vi "MeasEngine.vi"() -> (1 "XY graph visual":cluster{dbl[], dbl[]}(graph))   [LabVIEW 2026]
uses:
  <vilib>/Utility/miscctls.llb/LVRectTypeDef.ctl
  <vilib>/Utility/miscctls.llb/LVPointTypeDef.ctl
  <userlib>/Status.ctl
  <vilib>/Instr/_visa.llb/VISA Flush IO Buffer Mask.ctl
  <vilib>/Instr/_visa.llb/VISA Configure Serial Port (Instr).vi
  <vilib>/Analysis/3filter.llb/Butterworth Filter (DBL).vi
  <vilib>/measure/maspectr.llb/FFT Spectrum (Mag-Phase) for N Chan.vi
  <vilib>/measure/NI_MAPro.lvlib
  <vilib>/Analysis/NI_AALBase.lvlib
panel:
  in  "Okno osy X":dbl(slide) scale=5.0..30.0 scale format="%#_4g"
  in  "Cluster 2":T1={"Zařízení"="", "Cesta k uloženému souboru"=path "", "Vzorkovací frekvence"=enum."1000", "Record Button"=FALSE, "Stop Button"=FALSE, "A1 signál"=enum."EMG", "A2 signál"=enum."EMG", "A3 signál"=enum."EMG", "A4 signál"=enum."EMG", "A5 signál"=enum."EMG", "A6 signál"=enum."EMG", "Pin s připojeným signálem"=enum."A1"}
  in  "DO 2":bool
  in  "DO 1":bool
  out "Spectrum":cluster{"f0":dbl, "df":dbl, "magnitude":dbl[]}[](graph)
  in  "EditCluster":T2={"Horní mezní frekvence"=0.45000000000000007, "Dolní mezní frekvence"=0.0, "filter type"=enum."Lowpass", "applyFilter"=FALSE, "removeFilter"=FALSE, "undoFIlter"=FALSE} {"Horní mezní frekvence" format="%0.2f"}
  out "Waveform Graph Edit":waveform(dbl)[](graph)
  in  "DO 4":bool
  in  "DO 3":bool
  out "tdms file":refnum<k34>
  out "Ylabel and Plot name":cluster{string, string}
  out "Sample Rate Numeric":i32
  out "Consumer":i32
  out "producer":i32
  in  "error in (no error)":errorcluster
  out "Sync Stop":bool=TRUE
  # "Hz"
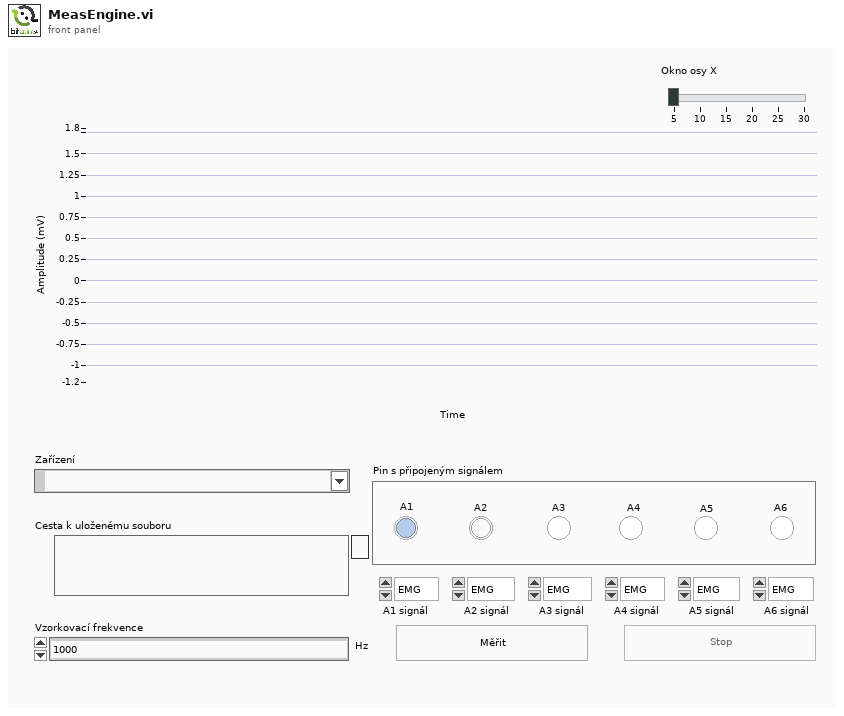
[diagram p1: front panel]
types:
  T1 = cluster{"Zařízení":refnum<visa-resource-name>, "Cesta k uloženému souboru":path, "Vzorkovací frekvence":enum16{"1", "10", "100", "1000"}, "Record Button":bool, "Stop Button":bool, "A1 signál":enum16{"EMG", "ECG", "EEG", "EDA", "ACC"}, "A2 signál":enum16{"EMG", "ECG", "EEG", "EDA", "ACC"}, "A3 signál":enum16{"EMG", "ECG", "EEG", "EDA", "ACC"}, "A4 signál":enum16{"EMG", "ECG", "EEG", "EDA", "ACC"}, "A5 signál":enum16{"EMG", "ECG", "EEG", "EDA", "ACC"}, "A6 signál":enum16{"EMG", "ECG", "EEG", "EDA", "ACC"}, "Pin s připojeným signálem":enum32{"A1", "A2", "A3", "A4", "A5", "A6"}}
  T2 = cluster{"Horní mezní frekvence":dbl, "Dolní mezní frekvence":dbl, "filter type":enum32{"Lowpass", "Highpass", "Bandpass", "Bandstop"}, "applyFilter":bool, "removeFilter":bool, "undoFIlter":bool}
  T3 = typedef "Status.ctl" = enum16{"Initialize", "Edit", "Standby", "Recording", "Exit"}
  T4 = enum16{"Always On", "Always Off", "Off While Running"}
  T5 = typedef "LVPointTypeDef.ctl" = cluster{"Horizontal":i16, "Vertical":i16}
  T6 = typedef "LVRectTypeDef.ctl" = cluster{"Left":i16, "Top":i16, "Right":i16, "Bottom":i16}
  T7 = enum8{"Enabled", "Disabled", "Disabled and Grayed Out"}
  T8 = enum16{"open", "open or create", "create or replace", "create", "open (read-only)"}
  T9 = typedef "VISA Flush IO Buffer Mask.ctl" = u16
  T10 = enum32{"Lowpass", "Highpass", "Bandpass", "Bandstop"}
  T11 = cluster{"A1 signál":enum16{"EMG", "ECG", "EEG", "EDA", "ACC"}, "A2 signál":enum16{"EMG", "ECG", "EEG", "EDA", "ACC"}, "A3 signál":enum16{"EMG", "ECG", "EEG", "EDA", "ACC"}, "A4 signál":enum16{"EMG", "ECG", "EEG", "EDA", "ACC"}, "A5 signál":enum16{"EMG", "ECG", "EEG", "EDA", "ACC"}, "A6 signál":enum16{"EMG", "ECG", "EEG", "EDA", "ACC"}}
  T12 = cluster{"Result":dbl, "Result":dbl, "Result":dbl, "Result":dbl, "Result":dbl, "Result":dbl}
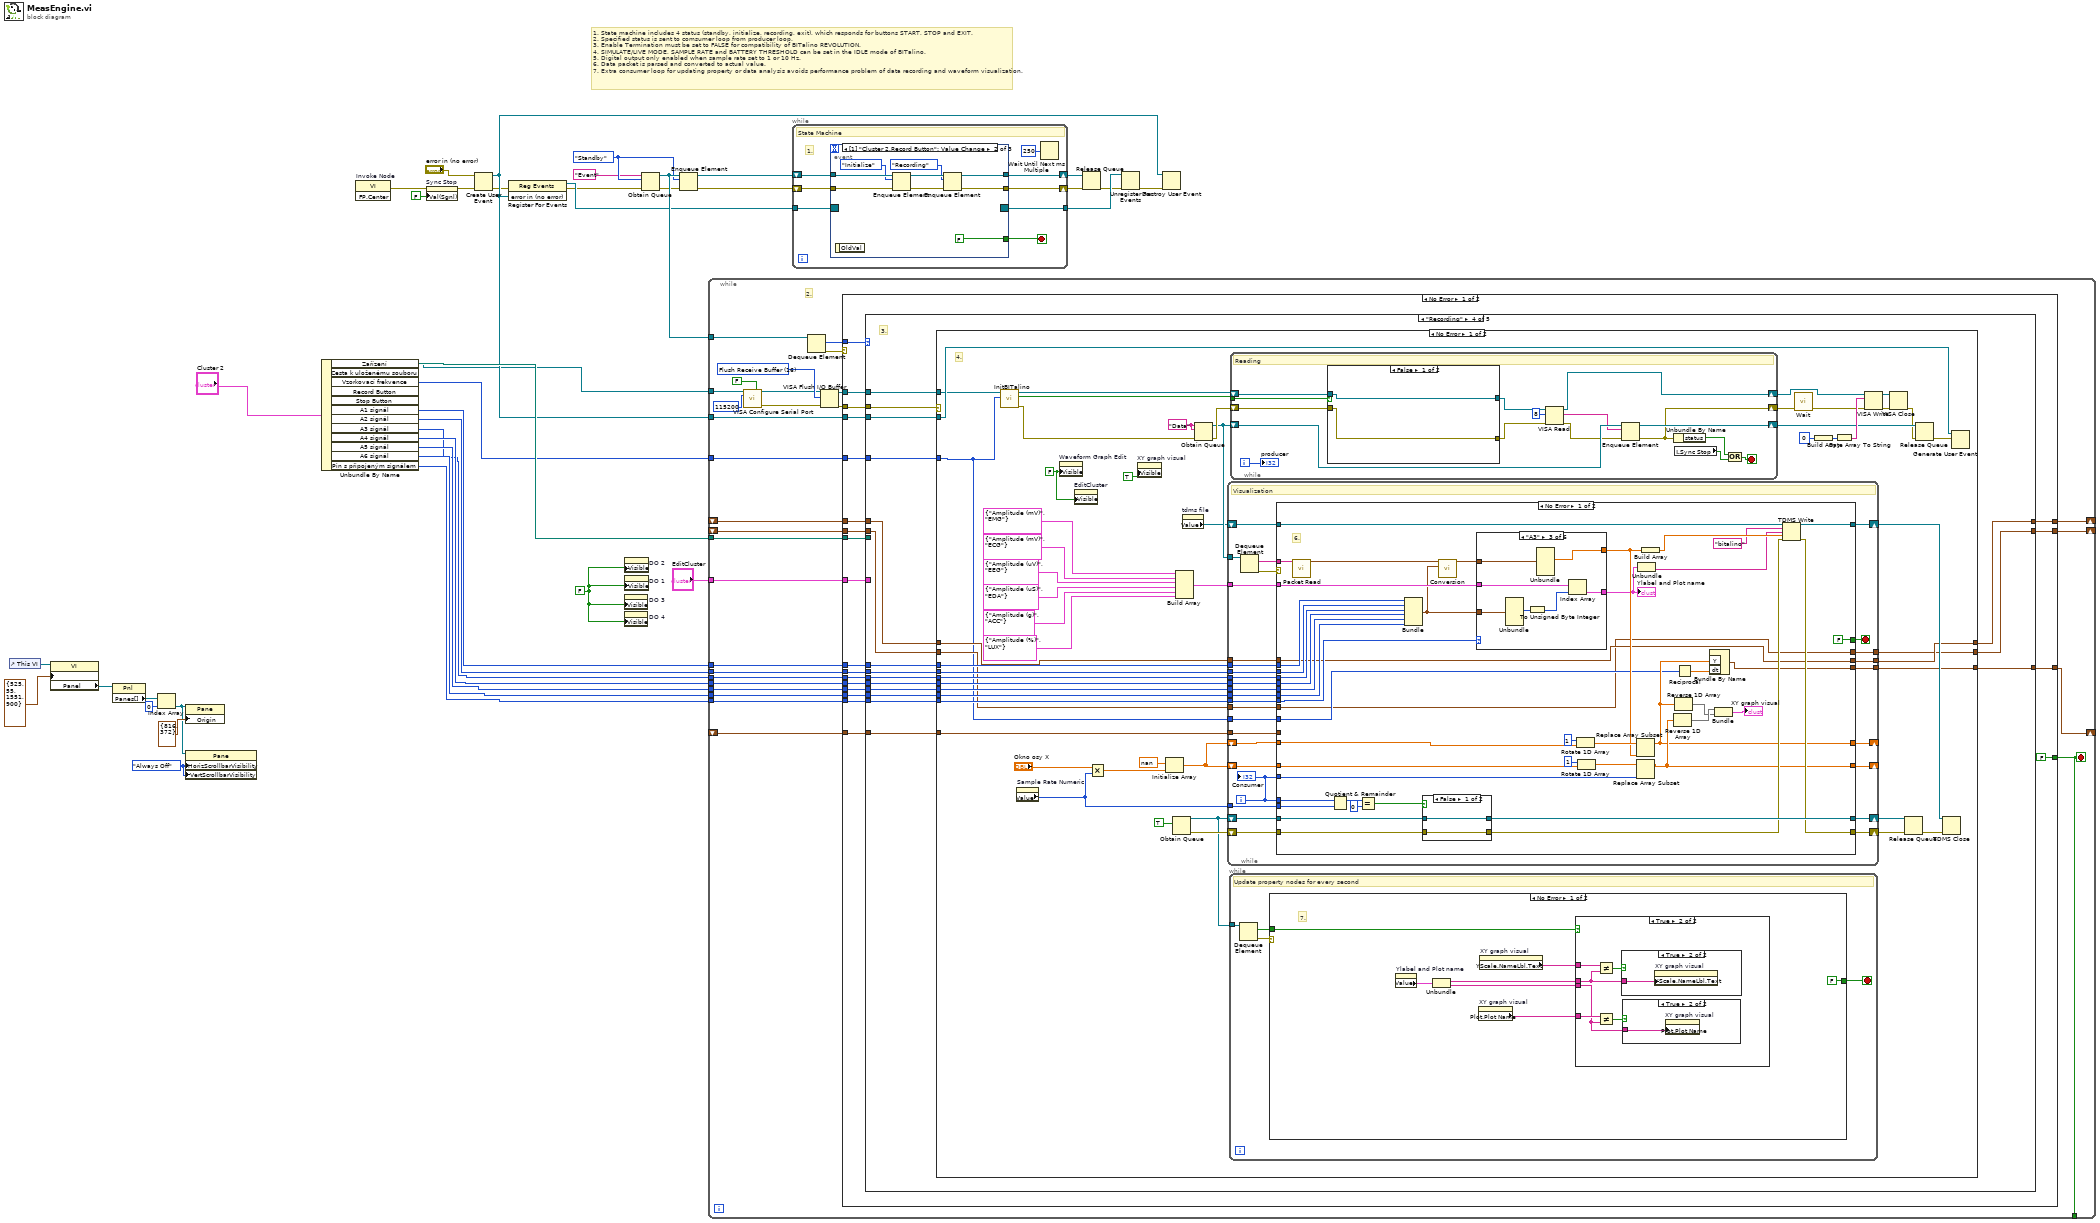
[diagram p0: block diagram]
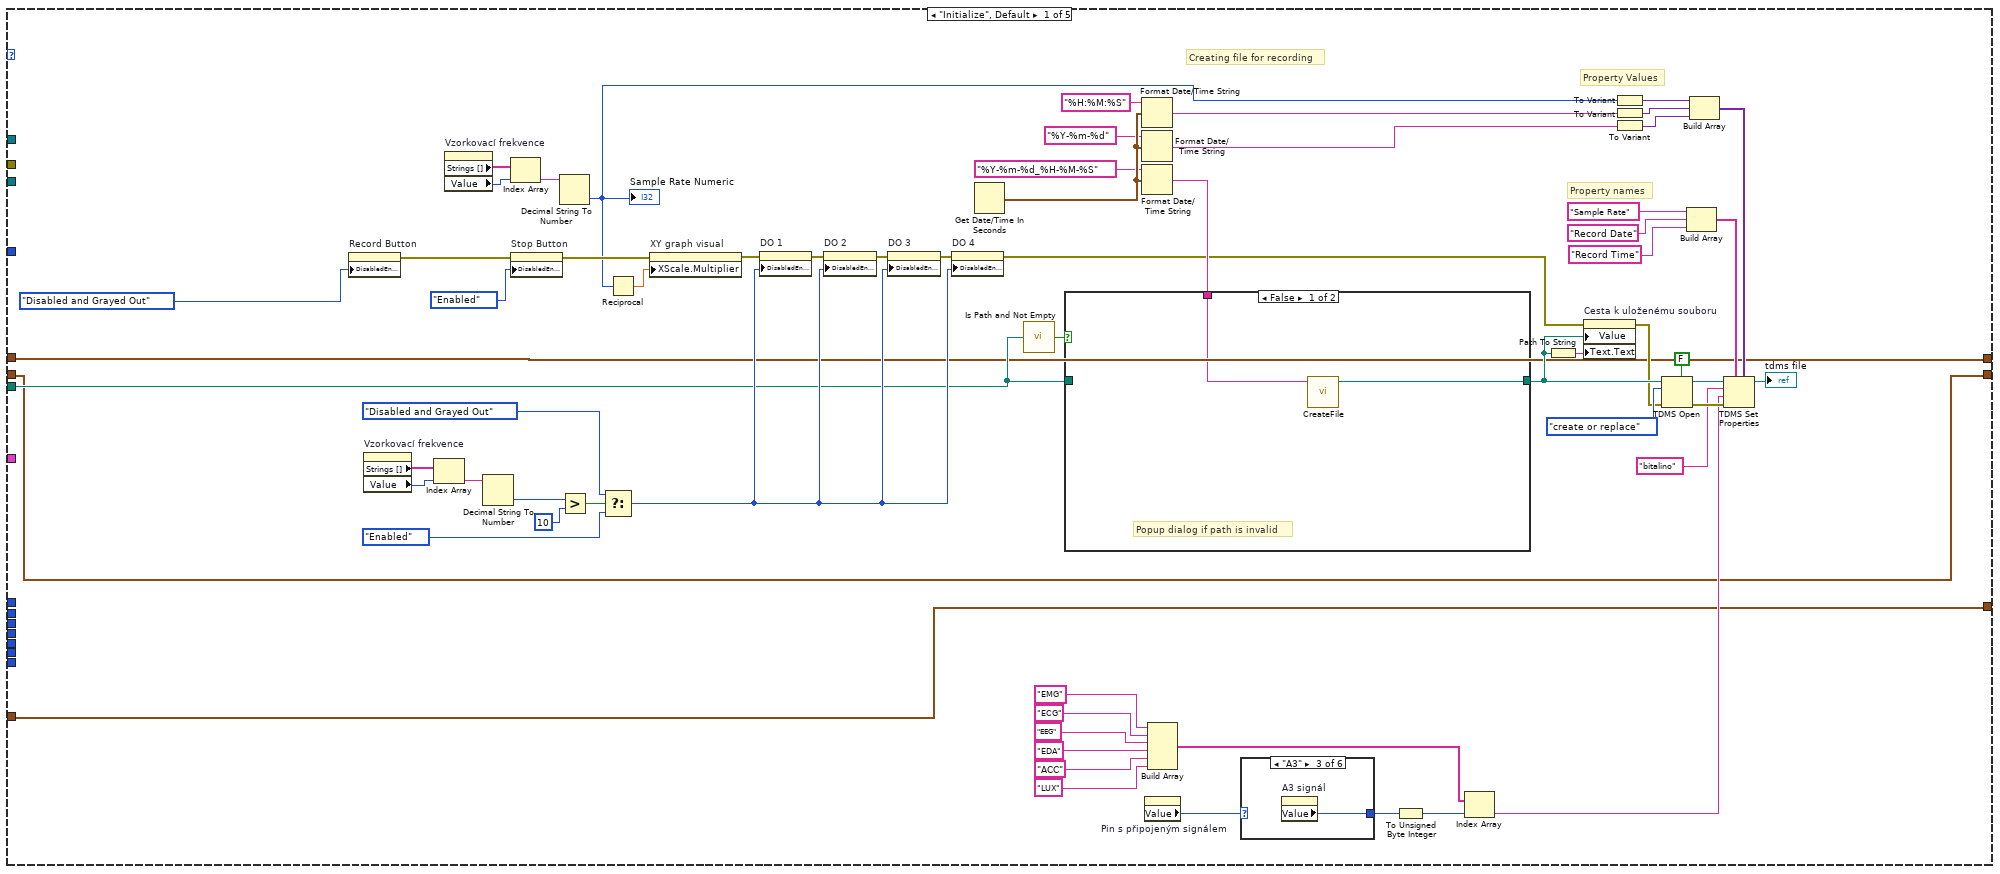
[diagram p2: hidden frame]
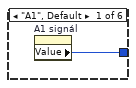
[diagram p3: hidden frame]
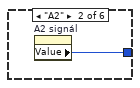
[diagram p4: hidden frame]
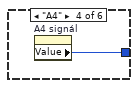
[diagram p5: hidden frame]
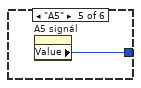
[diagram p6: hidden frame]
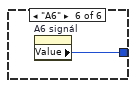
[diagram p7: hidden frame]
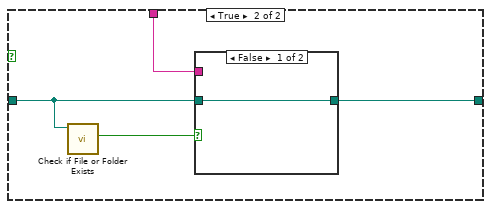
[diagram p8: hidden frame]
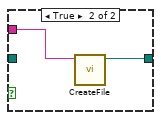
[diagram p9: hidden frame]
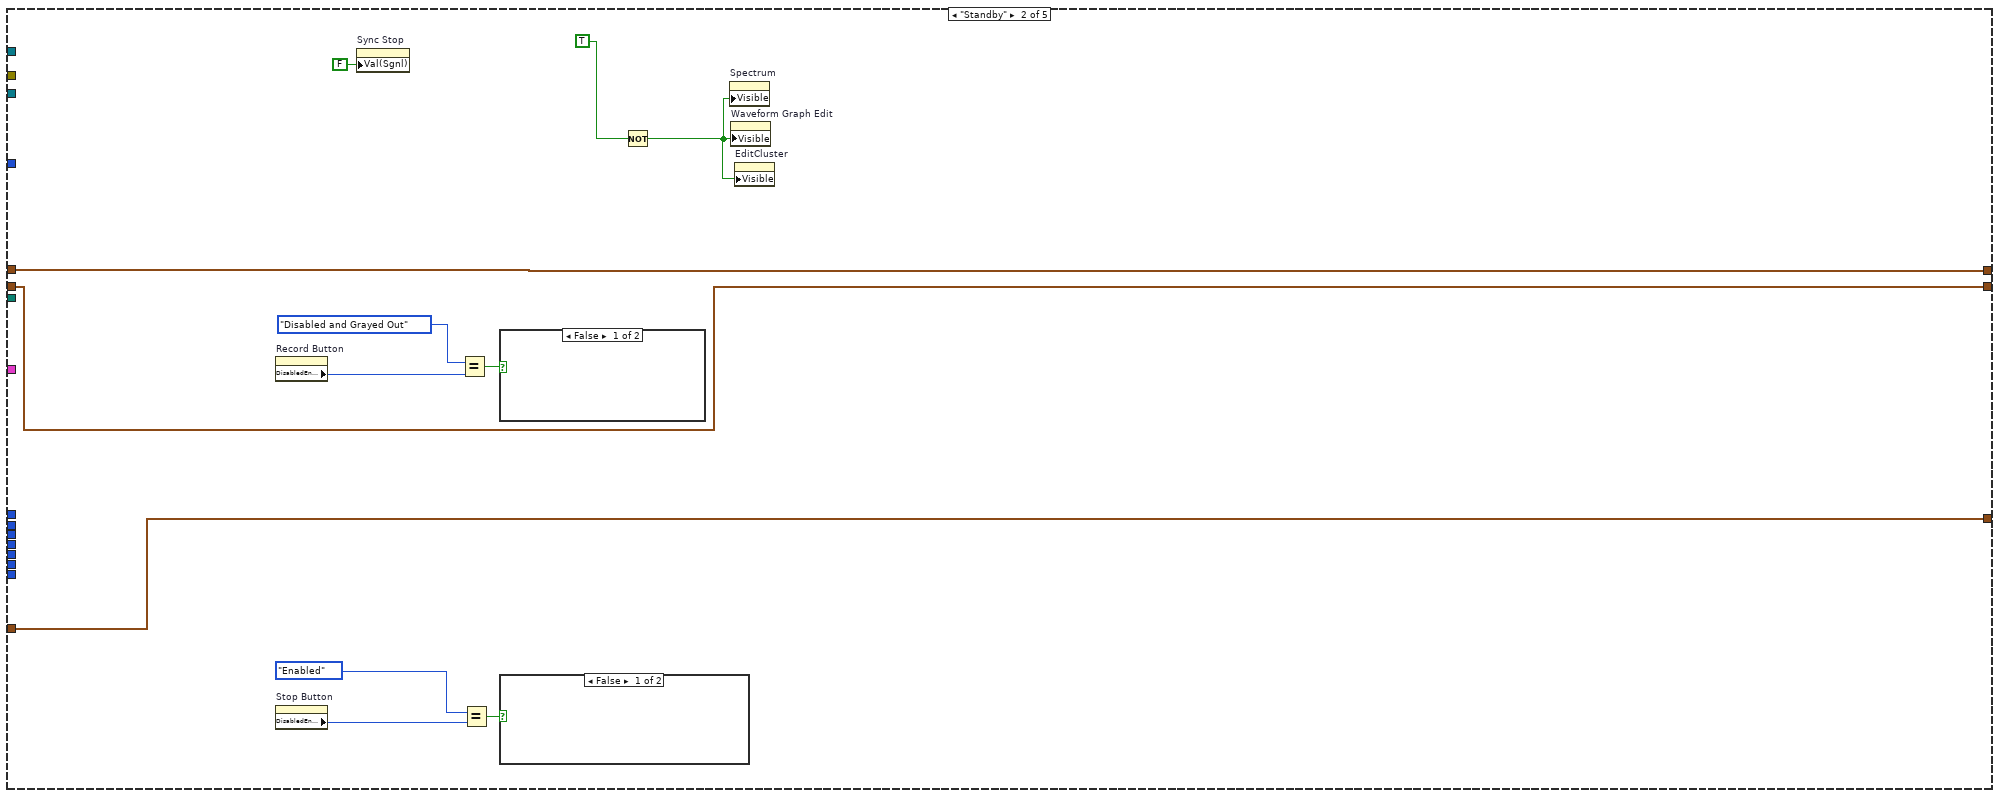
[diagram p10: hidden frame]
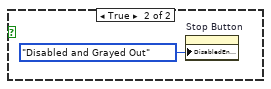
[diagram p11: hidden frame]
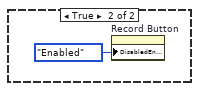
[diagram p12: hidden frame]
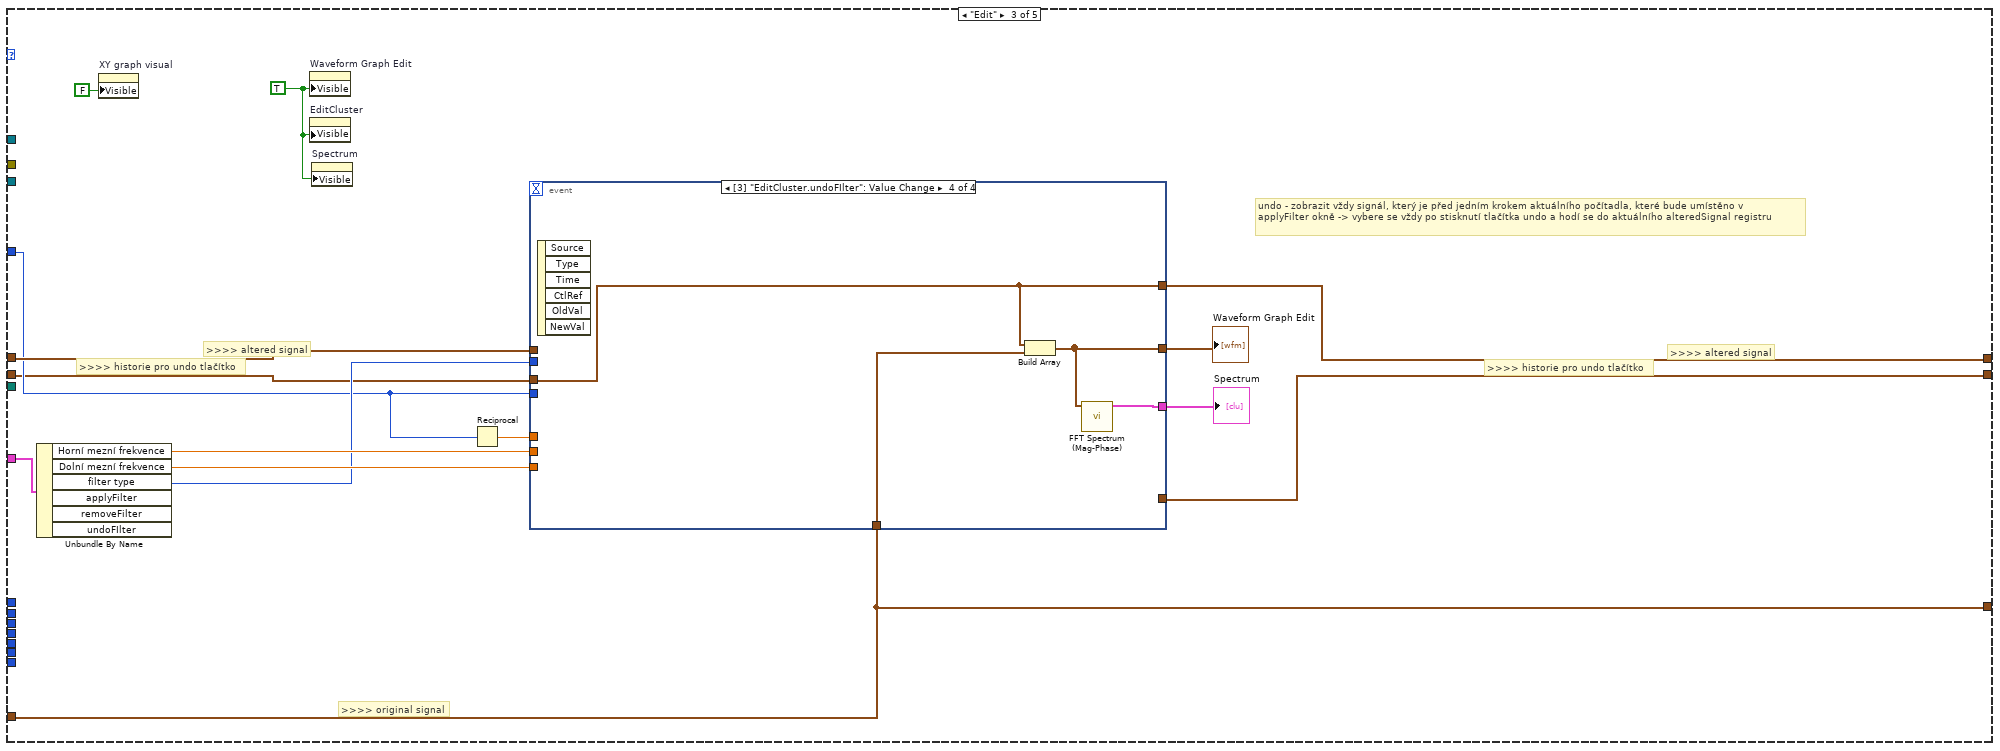
[diagram p13: hidden frame]
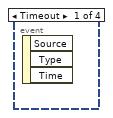
[diagram p14: hidden frame]
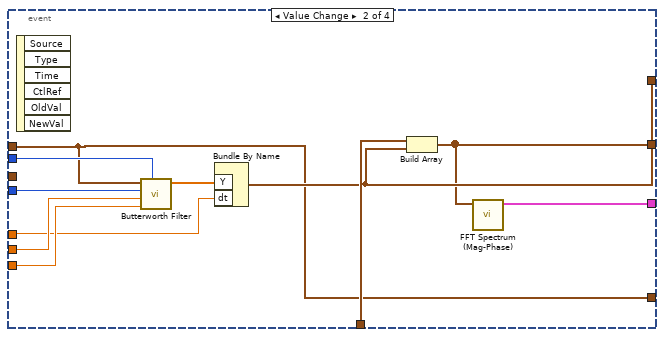
[diagram p15: hidden frame]
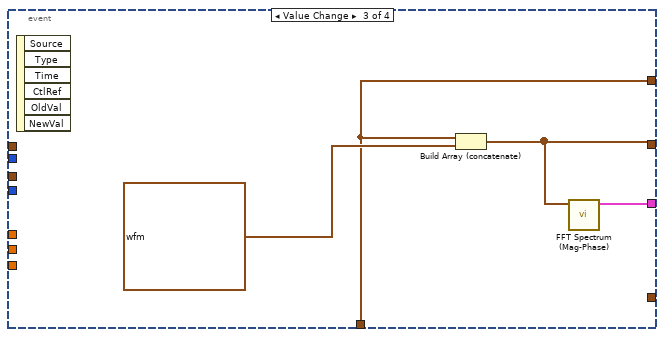
[diagram p16: hidden frame]
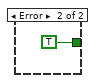
[diagram p20: hidden frame]
diagram:
  w5 = FALSE
  w3 = Status."Standby" ("Enum")
  w33 = T4."Always Off" ("Horizontal Scrollbar Visibility")
  # "1. State machine includes 4 status (standby, initialize, recording, exit), which responds for buttons START, STOP and EXIT.\n2. Specified status is sent to comsumer loop from producer loop.\n3. Enable Termination must be set to FALSE for compatibility of BITalino REVOLUTION.\n4. SIMULATE/LIVE MODE, SAMPLE RATE and BATTERY THRESHOLD can be set in the IDLE mode of BITalino.\n5. Digital output only enabled when sample rate set to 1 or 10 Hz.\n6. Data packet is parsed and converted to actual value.\n7. Extra consumer loop for updating property or data analysis avoids performance problem of data recording and waveform visualization."
  n1 = control-ref of="This VI"() -> (w40:refnum<vi>)
  n2 = property class="VI"(reference=w40, "Front Panel.WinBounds"=T6 {"Left"=525, "Top"=55, "Right"=1551, "Bottom"=900} ("Front Panel Window:Window Bounds")) -> ("Panel"=w38:refnum<vi>)  [unwired: 1 in, 2 out]
  n3 = property class="Pnl"(reference=w38) -> ("Panes[]"=w37:refnum<vi>[])  [unwired: 1 in, 2 out]
  n4 = Index Array(array=w37, index=0) -> (element=w34:refnum<vi>)
  n5 = property class="Pane"(reference=w34, "Origin"=T5 {"Horizontal"=816, "Vertical"=372}) -> ()  [unwired: 1 in, 2 out]
  n6 = property class="Pane"(reference=w34, "HorizScrollbarVisibility"=w33, "VertScrollbarVisibility"=w33) -> ()  [unwired: 1 in, 2 out]
  n7 = Unbundle By Name("Cluster 2") -> ("Zařízení"=w1:refnum<visa-resource-name>, "Cesta k uloženému souboru"=w30:path, "Vzorkovací frekvence"=w22:enum16{"1", "10", "100", "1000"}, "A1 signál"=w23:enum16{"EMG", "ECG", "EEG", "EDA", "ACC"}, "A2 signál"=w24:enum16{"EMG", "ECG", "EEG", "EDA", "ACC"}, "A3 signál"=w25:enum16{"EMG", "ECG", "EEG", "EDA", "ACC"}, "A4 signál"=w26:enum16{"EMG", "ECG", "EEG", "EDA", "ACC"}, "A5 signál"=w27:enum16{"EMG", "ECG", "EEG", "EDA", "ACC"}, "A6 signál"=w28:enum16{"EMG", "ECG", "EEG", "EDA", "ACC"}, "Pin s připojeným signálem"=w29:enum32{"A1", "A2", "A3", "A4", "A5", "A6"})  [unwired: 2 out]
  n8 = invoke on="Invoke Node" class="VI" method="FP.Center"() -> (error out=w20:errorcluster)  [unwired: 3 in, 2 out]
  n9 = property on="Sync Stop" class="Bool (strict)"(error in=w20, "Val(Sgnl)"=FALSE ("Value (Signaling)")) -> (error out=w11:errorcluster)  [unwired: 1 in, 1 out]
  n10 = Create User Event(user event datatype="error in (no error)", error in=w11) -> (user event=w19:refnum<user-event>, error out=w12:errorcluster)
  n11 = register-events(error in=w12, w19) -> (reference out=w14:refnum<event-registration>, error out=w13:errorcluster)  [unwired: 1 in]
  n12 = property on="DO 3" class="Bool (strict)"("Visible"=w5) -> ()  [unwired: 2 in, 2 out]
  n13 = property on="DO 4" class="Bool (strict)"("Visible"=w5) -> ()  [unwired: 2 in, 2 out]
  n14 = property on="DO 2" class="Bool (strict)"("Visible"=w5) -> ()  [unwired: 2 in, 2 out]
  n15 = property on="DO 1" class="Bool (strict)"("Visible"=w5) -> ()  [unwired: 2 in, 2 out]
  n16 = Obtain Queue(name (unnamed)="Event", element data type=w3, error in (no error)=w13) -> (queue out=w21:refnum<queue>, error out=w8:errorcluster)  [unwired: 2 in, 1 out]
  n17 = Enqueue Element(queue=w21, element=w3, error in (no error)=w8) -> (queue out=w10:refnum<queue>, error out=w9:errorcluster)  [unwired: 1 in, 1 out]
  n18 = while {
    tunnel: w21 -> [w69]
    tunnel: w19 -> [w49]
    tunnel: w22 -> [w66]
    tunnel: [w65] -> _
    tunnel: w23 -> [w64]
    tunnel: w24 -> [w63]
    tunnel: w25 -> [w62]
    tunnel: w26 -> [w61]
    tunnel: w27 -> [w60]
    tunnel: w28 -> [w59]
    tunnel: w29 -> [w58]
    tunnel: w30 -> [w57]
    shift-right: [w56] -> _
    shift-left: _ -> [w55]
    tunnel: "EditCluster" -> [w54]
    shift-right: [w53] -> _
    shift-left: _ -> [w52]
    shift-right: [w51] -> _
    shift-left: _ -> [w50]
    tunnel: w1 -> [w45]
    stop <- w65 stop-if-true
    w46 = T9 16 items=["Flush Receive Buffer"=16, "Write Transmit Buffer to Device"=32, "Flush Receive Buffer (No I/O)"=64, "Flush Transmit Buffer"=128] ("Mask")
    # "2."
    n19 = call-poly "VISA Configure Serial Port"("VISA resource name"=w45, "Enable Termination\nChar (T)"=FALSE ("Enable Termination\nChar (T)"), "baud rate (9600)"=u32 115200) -> ("VISA resource name out"=w42:refnum<visa-resource-name>, "error out"=w41:errorcluster)  [unwired: 11 in]
    n20 = Dequeue Element(queue=w69) -> (element=w68:T3, error out=w67:errorcluster)  [unwired: 2 in, 2 out]
    n21 = VISA Flush I/O Buffer(VISA resource name=w42, mask (16)=w46, error in (no error)=w41) -> (VISA resource name out=w47:refnum<visa-resource-name>, error out=w48:errorcluster)
    n22 = case shown="No Error" w67 {
      tunnel: w68 -> [w88 _]
      tunnel: [FALSE TRUE] -> w65
      tunnel: w66 -> [w89 _]
      tunnel: w64 -> [w87 _]
      tunnel: w63 -> [w86 _]
      tunnel: w62 -> [w85 _]
      tunnel: w61 -> [w84 _]
      tunnel: w60 -> [w83 _]
      tunnel: w59 -> [w82 _]
      tunnel: w58 -> [w81 _]
      tunnel: w57 -> [w80 _]
      tunnel: [w79 w484] -> w56
      tunnel: w55 -> [w78 w484]
      tunnel: w54 -> [w77 _]
      tunnel: [w76 w483] -> w53
      tunnel: w52 -> [w75 w483]
      tunnel: [w74 w482] -> w51
      tunnel: w50 -> [w73 w482]
      tunnel: w49 -> [w72 _]
      tunnel: w48 -> [w71 _]
      tunnel: w47 -> [w70 _]
      frame No Error {
        n23 = case shown="\"Recording\"" w88 {
          tunnel: w89 -> [_ _ w189 w233 _]
          tunnel: w87 -> [_ _ _ w232 _]
          tunnel: w86 -> [_ _ _ w231 _]
          tunnel: w85 -> [_ _ _ w230 _]
          tunnel: w84 -> [_ _ _ w229 _]
          tunnel: w83 -> [_ _ _ w228 _]
          tunnel: w82 -> [_ _ _ w227 _]
          tunnel: w81 -> [_ _ _ w226 _]
          tunnel: w80 -> [w95 _ _ _ _]
          tunnel: [w94 w173 w186 w225 w479] -> w79
          tunnel: w78 -> [w94 w173 w186 w224 w479]
          tunnel: w77 -> [_ _ w196 _ _]
          tunnel: [w93 w169 w185 w223 w478] -> w76
          tunnel: w75 -> [w93 w169 w194 w222 w478]
          tunnel: [w92 w171 w184 w221 w477] -> w74
          tunnel: w73 -> [w92 w171 w183 w220 w477]
          tunnel: w72 -> [_ _ _ w219 _]
          tunnel: w71 -> [_ _ _ w218 _]
          tunnel: w70 -> [_ _ _ w217 _]
          frame "Initialize", Default {
            # "Creating file for recording"
            # "Property Values"
            # "Property names"
            n24 = property on="Record Button" class="Bool"("DisabledEnum"=T7."Disabled and Grayed Out" ("Disabled")) -> (error out=w91:errorcluster)  [unwired: 2 in, 1 out]
            n25 = property on="Vzorkovací frekvence" class="Enum (strict)"() -> ("Strings []"=w113:string[], "Value"=w112:enum16{"1", "10", "100", "1000"})  [unwired: 2 in, 2 out]
            n26 = Index Array "Index Array"(array=w113, index=w112) -> (element=w111:string)
            n27 = property on="Vzorkovací frekvence" class="Enum (strict)"() -> ("Strings []"=w152:string[], "Value"=w151:enum16{"1", "10", "100", "1000"})  [unwired: 2 in, 2 out]
            n28 = Decimal String To Number(string=w111) -> (number=w110:i32)  [unwired: 2 in, 1 out]
            n29 = Index Array(array=w152, index=w151) -> (element=w150:string)
            n30 = property on="Stop Button" class="Bool"(error in=w91, "DisabledEnum"=T7."Enabled" ("Disabled")) -> (error out=w149:errorcluster)  [unwired: 1 in, 1 out]
            n31 = Decimal String To Number(string=w150) -> (number=w122:i32)  [unwired: 2 in, 1 out]
            "Sample Rate Numeric" <- w122
            n32 = Greater?(x=w110, y=10) -> (0:w118:bool)
            n33 = Select(t=T7."Disabled and Grayed Out" ("Disabled"), s=w118, f=T7."Enabled" ("Disabled")) -> (s? t:f=w121:T7)
            n34 = Reciprocal(x=w122) -> (1/x=w148:dbl)
            n35 = property on="XY graph visual" class="XYGraph (strict)"(error in=w149, "XScale.Multiplier"=w148) -> (error out=w109:errorcluster)  [unwired: 1 in, 1 out]
            n36 = property on="DO 1" class="Bool (strict)"(error in=w109, "DisabledEnum"=w121) -> (error out=w116:errorcluster)  [unwired: 1 in, 1 out]
            n37 = property on="DO 2" class="Bool (strict)"(error in=w116, "DisabledEnum"=w121) -> (error out=w115:errorcluster)  [unwired: 1 in, 1 out]
            n38 = property on="DO 3" class="Bool (strict)"(error in=w115, "DisabledEnum"=w121) -> (error out=w114:errorcluster)  [unwired: 1 in, 1 out]
            n39 = property on="DO 4" class="Bool (strict)"(error in=w114, "DisabledEnum"=w121) -> (error out=w108:errorcluster)  [unwired: 1 in, 1 out]
            n40 = Get Date/Time In Seconds() -> (seconds since 1Jan1904=w138:timestamp)
            n41 = call <vilib>:"Is Path and Not Empty.vi"("path"=w95) -> ("Is Path and Not Empty?"=w130:bool)  [unwired: 4 in]
            n42 = Format Date/Time String(time format string (%c)="%H:%M:%S", seconds (now)=w138) -> (date/time string=w143:string)  [unwired: 1 in]
            n43 = Format Date/Time String(time format string (%c)="%Y-%m-%d", seconds (now)=w138) -> (date/time string=w144:string)  [unwired: 1 in]
            n44 = Format Date/Time String(time format string (%c)="%Y-%m-%d_%H-%M-%S", seconds (now)=w138) -> (date/time string=w134:string)  [unwired: 1 in]
            n45 = case shown="False" w130 {
              tunnel: [w160 w163] -> w127
              tunnel: w95 -> [_ w162]
              tunnel: w134 -> [w161 w164]
              frame False {
                # "Popup dialog if path is invalid"
                n46 = call "CreateFile.vi"("date/time string"=w161) -> ("appended path"=w160:path)  [unwired: 10 in]
              }
              frame True {
                n47 = call <vilib>:"Check if File or Folder Exists.vi"("path"=w162) -> ("file or folder exists?"=w165:bool)  [unwired: 8 in, 2 out]
                n48 = case shown="False" w165 {
                  tunnel: w164 -> [_ w168]
                  tunnel: [w166 w167] -> w163
                  tunnel: w162 -> [w166 _]
                  frame False {
                  }
                  frame True {
                    n49 = call "CreateFile.vi"("date/time string"=w168) -> ("appended path"=w167:path)  [unwired: 10 in]
                  }
                }
              }
            }
            n50 = property on="Pin s připojeným signálem" class="RadioBtnsControl (strict)"() -> ("Value"=w106:enum32{"A1", "A2", "A3", "A4", "A5", "A6"})  [unwired: 2 in, 2 out]
            n51 = Build Array("EMG", "ECG", "EEG", "EDA", "ACC", "LUX") -> (w97:string[])
            n52 = case shown="\"A3\"" w106 {
              tunnel: [w154 w155 w156 w157 w158 w159] -> w99
              frame "A1", Default {
                n53 = property on="A1 signál" class="Enum (strict)"() -> ("Value"=w154:enum16{"EMG", "ECG", "EEG", "EDA", "ACC"})  [unwired: 2 in, 2 out]
              }
              frame "A2" {
                n54 = property on="A2 signál" class="Enum (strict)"() -> ("Value"=w155:enum16{"EMG", "ECG", "EEG", "EDA", "ACC"})  [unwired: 2 in, 2 out]
              }
              frame "A3" {
                n55 = property on="A3 signál" class="Enum (strict)"() -> ("Value"=w156:enum16{"EMG", "ECG", "EEG", "EDA", "ACC"})  [unwired: 2 in, 2 out]
              }
              frame "A4" {
                n56 = property on="A4 signál" class="Enum (strict)"() -> ("Value"=w157:enum16{"EMG", "ECG", "EEG", "EDA", "ACC"})  [unwired: 2 in, 2 out]
              }
              frame "A5" {
                n57 = property on="A5 signál" class="Enum (strict)"() -> ("Value"=w158:enum16{"EMG", "ECG", "EEG", "EDA", "ACC"})  [unwired: 2 in, 2 out]
              }
              frame "A6" {
                n58 = property on="A6 signál" class="Enum (strict)"() -> ("Value"=w159:enum16{"EMG", "ECG", "EEG", "EDA", "ACC"})  [unwired: 2 in, 2 out]
              }
            }
            n59 = To Unsigned Byte Integer(number=w99) -> (unsigned 8bit integer=w98:u8)
            n60 = Index Array(array=w97, index=w98) -> (element=w96:string)
            n61 = Path To String(path=w127) -> (string=w128:string)
            n62 = property on="Cesta k uloženému souboru" class="Path"(error in=w108, "Value"=w127, "Text.Text"=w128) -> (error out=w126:errorcluster)  [unwired: 1 in, 1 out]
            n63 = To Variant(anything=w122) -> (Variant=w142:variant)
            n64 = To Variant(anything=w143) -> (Variant=w145:variant)
            n65 = To Variant(anything=w144) -> (Variant=w146:variant)
            n66 = TDMS Open(5:FALSE ("create index file? (T)"), 8:w126, 10:T8."create or replace" ("operation (0:open)"), 11:w127) -> (0:w133:errorcluster, 3:w132:refnum<k34>)  [unwired: 3 in]
            n67 = Build Array("Sample Rate", "Record Date", "Record Time") -> (w141:string[])
            n68 = Build Array(w142, w145, w146) -> (w147:variant[])
            n69 = TDMS Set Properties(5:w147, 7:w141, 8:w133, 9:w96, 10:"bitalino", 11:w132) -> (3:→"tdms file":refnum<k34>)  [unwired: 3 out]
          }
          frame "Standby" {
            n70 = property on="Record Button" class="Bool"() -> ("DisabledEnum"=w179:T7)  [unwired: 2 in, 2 out]
            n71 = property on="Stop Button" class="Bool"() -> ("DisabledEnum"=w176:T7)  [unwired: 2 in, 2 out]
            n72 = property on="Sync Stop" class="Bool (strict)"("Val(Sgnl)"=FALSE ("Value (Signaling)")) -> ()  [unwired: 2 in, 2 out]
            n73 = Equal?(x=T7."Disabled and Grayed Out" ("Disabled"), y=w179) -> (x = y?=w178:bool)
            n74 = Equal?(x=T7."Enabled" ("Disabled"), y=w176) -> (x = y?=w175:bool)
            n75 = case shown="False" w178 {
              frame False {
              }
              frame True {
                n76 = property on="Record Button" class="Bool"("DisabledEnum"=T7."Enabled" ("Disabled")) -> ()  [unwired: 2 in, 2 out]
              }
            }
            n77 = case shown="False" w175 {
              frame False {
              }
              frame True {
                n78 = property on="Stop Button" class="Bool"("DisabledEnum"=T7."Disabled and Grayed Out" ("Disabled")) -> ()  [unwired: 2 in, 2 out]
              }
            }
            n79 = Not(x=TRUE ("Visible")) -> (.not. x?=w172:bool)
            n80 = property on="Spectrum" class="WFGraph (strict)"("Visible"=w172) -> ()  [unwired: 2 in, 2 out]
            n81 = property on="Waveform Graph Edit" class="WFGraph (strict)"("Visible"=w172) -> ()  [unwired: 2 in, 2 out]
            n82 = property on="EditCluster" class="Clust"("Visible"=w172) -> ()  [unwired: 2 in, 2 out]
          }
          frame "Edit" {
            w195 = TRUE ("Visible")
            # ">>>> altered signal"
            # ">>>> historie pro undo tlačítko"
            # ">>>> historie pro undo tlačítko"
            # "undo - zobrazit vždy signál, který je před jedním krokem aktuálního počítadla, které bude umístěno v \napplyFilter okně -> vybere se vždy po stisknutí tlačítka undo a hodí se do aktuálního alteredSignal registru"
            # ">>>> altered signal"
            # ">>>> original signal"
            n83 = Unbundle By Name(w196) -> ("Horní mezní frekvence"=w192:dbl, "Dolní mezní frekvence"=w191:dbl, "filter type"=w190:T10)  [unwired: 3 out]
            n84 = property on="XY graph visual" class="XYGraph (strict)"("Visible"=FALSE) -> ()  [unwired: 2 in, 2 out]
            n85 = property on="Waveform Graph Edit" class="WFGraph (strict)"("Visible"=w195) -> ()  [unwired: 2 in, 2 out]
            n86 = property on="EditCluster" class="Clust"("Visible"=w195) -> ()  [unwired: 2 in, 2 out]
            n87 = property on="Spectrum" class="WFGraph (strict)"("Visible"=w195) -> ()  [unwired: 2 in, 2 out]
            n88 = Reciprocal(x=w189) -> (1/x=w193:dbl)
            n89 = event shown="[3] \"EditCluster.undoFIlter\": Value Change" {
              selector: _ -> [_ _ _ _]
              dyn-events: _ -> [_ _ _ _]
              timeout: _ -> [_ _ _ _]
              tunnel: w186 -> [_ w207 w209 w215]
              tunnel: [_ w206 w209 w216] -> w185
              tunnel: w194 -> [_ w198 _ _]
              tunnel: w193 -> [_ w202 _ _]
              tunnel: w192 -> [_ w205 _ _]
              tunnel: w191 -> [_ w204 _ _]
              tunnel: w190 -> [_ w203 _ _]
              tunnel: w189 -> [_ w201 _ _]
              tunnel: [_ w200 w210 w213] -> w188
              tunnel: [_ w199 w211 w214] -> w187
              tunnel: [_ w198 _ _] -> w184
              tunnel: w183 -> [_ _ _ w216]
              event Timeout {
                n90 = event-data() -> ()  [unwired: 1 in, 3 out]
              }
              event "EditCluster.applyFilter": Value Change {
                n91 = event-data() -> ()  [unwired: 1 in, 6 out]
                n92 = call-poly <vilib>:"Butterworth Filter.vi"("filter type"=w203, "low cutoff freq: fl"=w204, "high cutoff freq: fh"=w205, "sampling freq: fs"=w201, "X"=w198) -> ("Filtered X"=w208:dbl[])  [unwired: 3 in, 1 out]
                n93 = Bundle By Name("Y"=w208, "dt"=w202) -> (w206:waveform(dbl))  [unwired: 1 in]
                n94 = Build Array(w207, w206) -> (w200:waveform(dbl)[])
                n95 = call-poly <vilib>:"FFT Spectrum (Mag-Phase).vi"("time signals"=w200) -> ("magnitudes"=w199:cluster{"f0":dbl, "df":dbl, "magnitude":dbl[]}[])  [unwired: 6 in, 4 out]
              }
              event "EditCluster.removeFilter": Value Change {
                n96 = event-data() -> ()  [unwired: 1 in, 6 out]
                n97 = Build Array (concatenate)(w209, waveform(dbl)[] [{"t0"=timestamp(-3600 s since 1904-01-01), "dt"=10000.0, "Y"=[0.0]}] ("array")) -> (w210:waveform(dbl)[])
                n98 = call-poly <vilib>:"FFT Spectrum (Mag-Phase).vi"("time signals"=w210) -> ("magnitudes"=w211:cluster{"f0":dbl, "df":dbl, "magnitude":dbl[]}[])  [unwired: 6 in, 4 out]
              }
              event "EditCluster.undoFIlter": Value Change {
                n99 = event-data() -> ()  [unwired: 1 in, 6 out]
                n100 = Build Array(w216, w215) -> (w213:waveform(dbl)[])
                n101 = call-poly <vilib>:"FFT Spectrum (Mag-Phase).vi"("time signals"=w213) -> ("magnitudes"=w214:cluster{"f0":dbl, "df":dbl, "magnitude":dbl[]}[])  [unwired: 6 in, 4 out]
              }
            }
            "Waveform Graph Edit" <- w188
            "Spectrum" <- w187
          }
          frame "Recording" {
            # "3."
            n102 = case shown="No Error" w218 {
              selector: w218 -> [_ w475]
              tunnel: w219 -> [w275 w476]
              tunnel: w233 -> [w236 _]
              tunnel: w232 -> [w254 _]
              tunnel: w231 -> [w253 _]
              tunnel: w230 -> [w252 _]
              tunnel: w229 -> [w251 _]
              tunnel: w228 -> [w250 _]
              tunnel: w227 -> [w249 _]
              tunnel: w226 -> [w248 _]
              tunnel: [w247 w474] -> w225
              tunnel: w224 -> [w245 w474]
              tunnel: [w244 w473] -> w223
              tunnel: w222 -> [w243 w473]
              tunnel: [w241 w472] -> w221
              tunnel: w220 -> [w240 w472]
              tunnel: w217 -> [w239 _]
              frame No Error {
                w242 = FALSE ("Visible")
                w283 = "Data"
                # "4."
                n103 = call "InitBITalino.vi"("Sample Rate"=w236, "BITalino"=w239) -> ("error out"=w235:errorcluster, "Digital Output"=w237:bool, "VISA out"=w238:refnum<visa-resource-name>)  [unwired: 7 in]
                n104 = property on="Sample Rate Numeric" class="DigNum (strict)"() -> ("Value"=w268:i32)  [unwired: 2 in, 2 out]
                n105 = property on="Waveform Graph Edit" class="WFGraph (strict)"("Visible"=w242) -> ()  [unwired: 2 in, 2 out]
                n106 = property on="EditCluster" class="Clust"("Visible"=w242) -> ()  [unwired: 2 in, 2 out]
                n107 = Multiply(x="Okno osy X", y=w268) -> (x*y=w266:dbl)
                n108 = property on="XY graph visual" class="XYGraph (strict)"("Visible"=TRUE) -> ()  [unwired: 2 in, 2 out]
                n109 = Initialize Array(nan ("element"), w266) -> (w265:dbl[])
                n110 = Obtain Queue(element data type=TRUE) -> (queue out=w271:refnum<queue>, error out=w273:errorcluster)  [unwired: 4 in, 1 out]
                n111 = Build Array(cluster{string, string} {"Amplitude (mV)", "EMG"}, cluster{string, string} {"Amplitude (mV)", "ECG"}, cluster{string, string} {"Amplitude (uV)", "EEG"}, cluster{string, string} {"Amplitude (uS)", "EDA"}, cluster{string, string} {"Amplitude (g)", "ACC"}, cluster{string, string} {"Amplitude (%)", "LUX"}) -> (w258:cluster{string, string}[])
                n112 = property on="tdms file" class="Ref (strict)"() -> ("Value"=w257:refnum<k34>)  [unwired: 2 in, 2 out]
                n113 = Obtain Queue(name (unnamed)=w283, element data type=w283, error in (no error)=w235) -> (queue out=w284:refnum<queue>, error out=w285:errorcluster)  [unwired: 2 in, 1 out]
                n114 = while {
                  tunnel: w284 -> [w339]
                  shift-right: [w334] -> _
                  shift-left: w265 -> [w335]
                  tunnel: w268 -> [w333]
                  shift-right: [w330] -> w270
                  shift-left: w271 -> [w332]
                  shift-right: [w329] -> w269
                  shift-left: w273 -> [w331]
                  shift-right: [w326] -> _
                  shift-left: w265 -> [w328]
                  tunnel: w258 -> [w325]
                  shift-right: [w323] -> w255
                  shift-left: w257 -> [w324]
                  tunnel: w254 -> [w322]
                  tunnel: w253 -> [w321]
                  tunnel: w252 -> [w320]
                  tunnel: w251 -> [w319]
                  tunnel: w250 -> [w318]
                  tunnel: w249 -> [w317]
                  tunnel: w248 -> [w316]
                  tunnel: w236 -> [w315]
                  tunnel: [w314] -> w247
                  tunnel: w245 -> [w313]
                  tunnel: [w312] -> w244
                  tunnel: w243 -> [w311]
                  tunnel: [w310] -> w241
                  tunnel: w240 -> [w309]
                  i -> [w327]
                  stop <- w337 stop-if-true
                  # "Visualization"
                  n115 = Dequeue Element(queue=w339) -> (element=w336:string, error out=w338:errorcluster)  [unwired: 2 in, 2 out]
                  n116 = case shown="No Error" w338 {
                    tunnel: [FALSE TRUE] -> w337
                    tunnel: w336 -> [w361 _]
                    tunnel: w335 -> [w374 w443]
                    tunnel: [w347 w443] -> w334
                    tunnel: w333 -> [w375 _]
                    tunnel: w327 -> [w380 _]
                    tunnel: w332 -> [w383 w442]
                    tunnel: w331 -> [w382 w441]
                    tunnel: [w381 w442] -> w330
                    tunnel: [w362 w441] -> w329
                    tunnel: w328 -> [w371 w440]
                    tunnel: w327 -> [w370 _]
                    tunnel: [w350 w440] -> w326
                    tunnel: w325 -> [w369 _]
                    tunnel: w324 -> [w367 w439]
                    tunnel: [w366 w439] -> w323
                    tunnel: w322 -> [w357 _]
                    tunnel: w321 -> [w356 _]
                    tunnel: w320 -> [w355 _]
                    tunnel: w319 -> [w354 _]
                    tunnel: w318 -> [w353 _]
                    tunnel: w317 -> [w352 _]
                    tunnel: w316 -> [w351 _]
                    tunnel: w315 -> [w345 _]
                    tunnel: [w344 w438] -> w314
                    tunnel: w313 -> [_ w438]
                    tunnel: [w343 w437] -> w312
                    tunnel: w311 -> [w343 w437]
                    tunnel: [w342 w436] -> w310
                    tunnel: w309 -> [w342 w436]
                    frame No Error {
                      # "6."
                      n117 = call "Packet Read.vi"("Packets"=w361) -> ("Analog Channels"=w360:cluster{u16, u16, u16, u16, u16, u16})  [unwired: 7 in, 3 out]
                      n118 = Quotient & Remainder(x=w380, y=w375) -> (x-y*floor(x/y)=w379:i32)  [unwired: 1 out]
                      n119 = Equal?(x=w379, y=0) -> (x = y?=w377:bool)
                      n120 = Bundle "Bundle"("A1 signál"=w357, "A2 signál"=w356, "A3 signál"=w355, "A4 signál"=w354, "A5 signál"=w353, "A6 signál"=w352) -> (w368:T11)  [unwired: 1 in]
                      n121 = case shown="False" w377 {
                        tunnel: w383 -> [w388 w393]
                        tunnel: w382 -> [w387 w392]
                        tunnel: [w388 w391] -> w381
                        tunnel: [w387 w390] -> w365
                        frame False {
                        }
                        frame True {
                          n122 = Enqueue Element(queue=w393, element=TRUE, error in (no error)=w392) -> (queue out=w391:refnum<queue>, error out=w390:errorcluster)  [unwired: 1 in, 1 out]
                        }
                      }
                      n123 = call "Conversion.vi"("Sensor Type"=w368, "Analog Channels"=w360) -> ("Converted Values"=w385:T12)  [unwired: 8 in, 1 out]
                      n124 = case shown="\"A3\"" w351 {
                        tunnel: w385 -> [w400 w407 w414 w421 w428 w435]
                        tunnel: [w399 w406 w413 w420 w427 w434] -> w364
                        tunnel: w369 -> [w395 w402 w409 w417 w423 w431]
                        tunnel: w368 -> [w398 w404 w411 w418 w425 w432]
                        tunnel: [w394 w401 w410 w416 w424 w430] -> w348
                        frame "A1", Default {
                          n125 = Unbundle(w398) -> ("A1 signál"=w396:enum16{"EMG", "ECG", "EEG", "EDA", "ACC"})  [unwired: 5 out]
                          n126 = To Unsigned Byte Integer(number=w396) -> (unsigned 8bit integer=w397:u8)
                          n127 = Unbundle(w400) -> ("Result"=w399:dbl)  [unwired: 5 out]
                          n128 = Index Array(array=w395, index=w397) -> (element=w394:cluster{string, string})
                        }
                        frame "A2" {
                          n129 = Unbundle(w404) -> ("A2 signál"=w403:enum16{"EMG", "ECG", "EEG", "EDA", "ACC"})  [unwired: 5 out]
                          n130 = To Unsigned Byte Integer(number=w403) -> (unsigned 8bit integer=w405:u8)
                          n131 = Unbundle(w407) -> ("Result"=w406:dbl)  [unwired: 5 out]
                          n132 = Index Array(array=w402, index=w405) -> (element=w401:cluster{string, string})
                        }
                        frame "A3" {
                          n133 = Unbundle(w411) -> ("A3 signál"=w408:enum16{"EMG", "ECG", "EEG", "EDA", "ACC"})  [unwired: 5 out]
                          n134 = To Unsigned Byte Integer(number=w408) -> (unsigned 8bit integer=w412:u8)
                          n135 = Unbundle(w414) -> ("Result"=w413:dbl)  [unwired: 5 out]
                          n136 = Index Array(array=w409, index=w412) -> (element=w410:cluster{string, string})
                        }
                        frame "A4" {
                          n137 = Unbundle(w418) -> ("A4 signál"=w415:enum16{"EMG", "ECG", "EEG", "EDA", "ACC"})  [unwired: 5 out]
                          n138 = To Unsigned Byte Integer(number=w415) -> (unsigned 8bit integer=w419:u8)
                          n139 = Unbundle(w421) -> ("Result"=w420:dbl)  [unwired: 5 out]
                          n140 = Index Array(array=w417, index=w419) -> (element=w416:cluster{string, string})
                        }
                        frame "A5" {
                          n141 = Unbundle(w425) -> ("A5 signál"=w422:enum16{"EMG", "ECG", "EEG", "EDA", "ACC"})  [unwired: 5 out]
                          n142 = Unbundle(w428) -> ("Result"=w427:dbl)  [unwired: 5 out]
                          n143 = To Unsigned Byte Integer(number=w422) -> (unsigned 8bit integer=w426:u8)
                          n144 = Index Array(array=w423, index=w426) -> (element=w424:cluster{string, string})
                        }
                        frame "A6" {
                          n145 = Unbundle(w432) -> ("A6 signál"=w429:enum16{"EMG", "ECG", "EEG", "EDA", "ACC"})  [unwired: 5 out]
                          n146 = To Unsigned Byte Integer(number=w429) -> (unsigned 8bit integer=w433:u8)
                          n147 = Unbundle(w435) -> ("Result"=w434:dbl)  [unwired: 5 out]
                          n148 = Index Array(array=w431, index=w433) -> (element=w430:cluster{string, string})
                        }
                      }
                      "Ylabel and Plot name" <- w348
                      n149 = Rotate 1D Array(1:w374, 2:1 ("n")) -> (0:w376:dbl[])
                      n150 = Rotate 1D Array(1:w371, 2:1 ("n")) -> (0:w372:dbl[])
                      n151 = Replace Array Subset(array=w376, new element=w364) -> (w347:dbl[])  [unwired: 1 in]
                      n152 = Replace Array Subset(array=w372, new element=w370) -> (w350:dbl[])  [unwired: 1 in]
                      n153 = Unbundle(w348) -> (w359:string)  [unwired: 1 out]
                      n154 = Build Array(w364) -> (w363:dbl[])
                      n155 = Reverse 1D Array(array=w350) -> (reversed array=w341:dbl[])
                      n156 = Reverse 1D Array(array=w347) -> (reversed array=w340:dbl[])
                      n157 = Reciprocal(x=w345) -> (1/x=w346:dbl)
                      n158 = Bundle By Name("Y"=w347, "dt"=w346) -> (w344:waveform(dbl))  [unwired: 1 in]
                      n159 = Bundle(w341, w340) -> (→"XY graph visual":cluster{dbl[], dbl[]})  [unwired: 1 in]
                      n160 = TDMS Write(0:w367, 5:"bitalino", 7:w359, 9:w363, 11:w365) -> (4:w366:refnum<k34>, 15:w362:errorcluster)  [unwired: 1 in, 2 out]
                    }
                    frame Error {
                    }
                  }
                  "Consumer" <- w327
                }
                n161 = while {
                  tunnel: w271 -> [w292]
                  stop <- w289 stop-if-true
                  # "Update property nodes for every second"
                  n162 = Dequeue Element(queue=w292) -> (element=w290:bool, error out=w291:errorcluster)  [unwired: 2 in, 2 out]
                  n163 = case shown="No Error" w291 {
                    tunnel: w290 -> [w296 _]
                    tunnel: [FALSE TRUE] -> w289
                    frame No Error {
                      # "7."
                      n164 = property on="Ylabel and Plot name" class="Clust (strict)"() -> ("Value"=w299:cluster{string, string})  [unwired: 2 in, 2 out]
                      n165 = Unbundle(w299) -> (w298:string, w297:string)
                      n166 = property on="XY graph visual" class="XYGraph (strict)"() -> ("Plot.Plot Name"=w293:string)  [unwired: 2 in, 2 out]
                      n167 = property on="XY graph visual" class="XYGraph (strict)"() -> ("YScale.NameLbl.Text"=w294:string)  [unwired: 2 in, 2 out]
                      n168 = case shown="True" w296 {
                        tunnel: w294 -> [_ w305]
                        tunnel: w293 -> [_ w301]
                        tunnel: w298 -> [_ w302]
                        tunnel: w297 -> [_ w300]
                        frame False {
                        }
                        frame True {
                          n169 = Not Equal?(x=w305, y=w302) -> (x != y?=w303:bool)
                          n170 = Not Equal?(x=w301, y=w300) -> (x != y?=w304:bool)
                          n171 = case shown="True" w303 {
                            tunnel: w302 -> [_ w307]
                            frame False {
                            }
                            frame True {
                              n172 = property on="XY graph visual" class="XYGraph (strict)"("YScale.NameLbl.Text"=w307) -> ()  [unwired: 2 in, 2 out]
                            }
                          }
                          n173 = case shown="True" w304 {
                            tunnel: w300 -> [_ w306]
                            frame False {
                            }
                            frame True {
                              n174 = property on="XY graph visual" class="XYGraph (strict)"("Plot.Plot Name"=w306) -> ()  [unwired: 2 in, 2 out]
                            }
                          }
                        }
                      }
                    }
                    frame Error {
                    }
                  }
                }
                n175 = while {
                  shift-right: [w458] -> w279
                  shift-left: w285 -> [w453]
                  shift-right: [w459] -> w282
                  shift-left: w284 -> [w460]
                  shift-right: [w445] -> w281
                  shift-left: w238 -> [w452]
                  tunnel: w237 -> [w451]
                  i -> [w457]
                  stop <- w456 stop-if-true
                  # "Reading"
                  n176 = case shown="False" w451 {
                    tunnel: w453 -> [w462 w468]
                    tunnel: w452 -> [w461 w467]
                    tunnel: [w462 w465] -> w449
                    tunnel: [w461 w466] -> w450
                    frame False {
                    }
                    frame True {
                      # "5."
                      n177 = call "Digital IO.vi"("DO 4"="DO 4", "DO 3"="DO 3", "DO in"="DO 2", "DO 1"="DO 1") -> ("string"=w471:string)
                      n178 = VISA Write(VISA resource name=w467, write buffer=w471, error in (no error)=w468) -> (VISA resource name out=w466:refnum<visa-resource-name>, error out=w465:errorcluster)  [unwired: 1 out]
                    }
                  }
                  n179 = VISA Read(VISA resource name=w450, byte count=u32 8, error in (no error)=w449) -> (VISA resource name out=w445:refnum<visa-resource-name>, read buffer=w447:string, error out=w448:errorcluster)  [unwired: 1 out]
                  n180 = Enqueue Element(queue=w460, element=w447, error in (no error)=w448) -> (queue out=w459:refnum<queue>, error out=w458:errorcluster)  [unwired: 1 in, 1 out]
                  n181 = Unbundle By Name(w458) -> ("status"=w454:bool)
                  n182 = local read "Sync Stop"() -> (w455:bool)
                  n183 = Compound Arithmetic op=OR(w454, w455) -> (w456:bool)
                  "producer" <- w457
                }
                n184 = call "Wait.vi"("error in (no error)"=w279) -> ("error out"=w280:errorcluster)  [unwired: 10 in]
                n185 = Build Array(u8 0) -> (w287:u8[])
                n186 = Byte Array To String(unsigned byte array=w287) -> (string=w286:string)
                n187 = VISA Write(VISA resource name=w281, write buffer=w286, error in (no error)=w280) -> (VISA resource name out=w277:refnum<visa-resource-name>, error out=w278:errorcluster)  [unwired: 1 out]
                n188 = VISA Close(VISA resource name=w277, error in (no error)=w278) -> (error out=w276:errorcluster)
                n189 = Release Queue(queue=w270, error in (no error)=w269) -> (error out=w256:errorcluster)  [unwired: 1 in, 2 out]
                n190 = Release Queue(queue=w282, error in (no error)=w276) -> (error out=w274:errorcluster)  [unwired: 1 in, 2 out]
                n191 = TDMS Close(8:w256, 11:w255) -> ()  [unwired: 2 out]
                n192 = Generate User Event(user event=w275, event data cluster=w274) -> ()  [unwired: 2 in, 2 out]
              }
              frame Error {
                n193 = Generate User Event(user event=w476, event data cluster=w475) -> ()  [unwired: 2 in, 2 out]
              }
            }
          }
          frame "Exit" {
            n194 = flat-sequence {
              frame #0 {
                n195 = property on="Stop Button" class="Bool"("DisabledEnum"=T7."Enabled" ("Disabled")) -> ()  [unwired: 2 in, 2 out]
              }
              frame #1 {
                n196 = Stop(stop? (T)=TRUE) -> ()
              }
            }
          }
        }
      }
      frame Error {
      }
    }
  }
  n197 = while {
    shift-right: [w490] -> w6
    shift-left: w10 -> [w493]
    shift-right: [w491] -> w7
    shift-left: w9 -> [w492]
    tunnel: w14 -> [w487]
    tunnel: [w486] -> w17
    stop <- w489 stop-if-true
    # "1."
    # "State Machine"
    n198 = event shown="[1] \"Cluster 2.Record Button\": Value Change" {
      selector: w487 -> [_ _ _]
      dyn-events: [_ _ _] -> w486
      timeout: _ -> [_ _ _]
      tunnel: w493 -> [w500 w510 w514]
      tunnel: w492 -> [w497 w509 w512]
      tunnel: [w494 w504 w511] -> w491
      tunnel: [w501 w506 w513] -> w490
      tunnel: [FALSE FALSE _] -> w489
      event "Cluster 2.Stop Button": Value Change {
        n199 = event-data() -> ()  [unwired: 1 in, 5 out]
        n200 = Enqueue Element(queue=w500, element=Status."Standby" ("Enum"), error in (no error)=w497) -> (queue out=w501:refnum<queue>, error out=w495:errorcluster)  [unwired: 1 in, 1 out]
        n201 = property on="Sync Stop" class="Bool (strict)"(error in=w495, "Val(Sgnl)"=TRUE) -> (error out=w494:errorcluster)  [unwired: 1 in, 1 out]
      }
      event "Cluster 2.Record Button": Value Change {
        n202 = event-data() -> ()  [unwired: 1 in, 1 out]
        n203 = Enqueue Element(queue=w510, element=Status."Initialize" ("Enum"), error in (no error)=w509) -> (queue out=w507:refnum<queue>, error out=w505:errorcluster)  [unwired: 1 in, 1 out]
        n204 = Enqueue Element(queue=w507, element=Status."Recording" ("Enum"), error in (no error)=w505) -> (queue out=w506:refnum<queue>, error out=w504:errorcluster)  [unwired: 1 in, 1 out]
      }
      event User Event {
        n205 = event-data() -> ()  [unwired: 1 in, 1 out]
        n206 = Enqueue Element(queue=w514, element=Status."Standby" ("Enum"), error in (no error)=w512) -> (queue out=w513:refnum<queue>, error out=w511:errorcluster)  [unwired: 1 in, 1 out]
      }
    }
    n207 = Wait Until Next ms Multiple(millisecond multiple=u32 250) -> ()  [unwired: 1 out]
  }
  n208 = Release Queue(queue=w6, error in (no error)=w7) -> (error out=w16:errorcluster)  [unwired: 1 in, 2 out]
  n209 = Unregister For Events(event registration refnum=w17, error in=w16) -> (error out=w18:errorcluster)
  n210 = Destroy User Event(user event=w19, error in=w18) -> ()  [unwired: 1 out]
